vi "PathVelocityProfile.vi"(0 "Pose":dbl[](array[numeric]), 1 "time":dbl, 3 "intervalo":dbl=0.016, 5 "estimatives":T1, 9 "Path  Smooth":dbl[][](array[numeric]), 11 "V_max":dbl format="%#_13g", 13 "Accel":dbl=10.0, 14 "DesAccel":dbl=15.0) -> (4 "Time X":dbl[](array[numeric]), 6 "Velocities X":dbl[](array[numeric]), 8 "Time Y":dbl[](array[numeric]), 10 "Velocities Y":dbl[](array[numeric]))   [LabVIEW 2023]
uses:
  Controle/VelocityProfileState.ctl
  Controls/estimatives.ctl
  <vilib>/Analysis/_algsub.llb/Real Vector Norm.vi
  <vilib>/Analysis/coordinate.llb/Wrap Angle (scalar).vi
  <vilib>/Analysis/NI_AAL_Angle.lvlib
  <vilib>/Analysis/NI_AALPro.lvlib
panel:
  in  "est_vy":dbl
  in  "est_vx":dbl
  out "VelocityProfile Y":T2[](array[typedef])
  out "VelocityProfile X":T2[](array[typedef])
  out "Velocity Profile Y":cluster{dbl[], dbl[]}[](graph)
  out "Velocity Profile X":cluster{dbl[], dbl[]}[](graph)
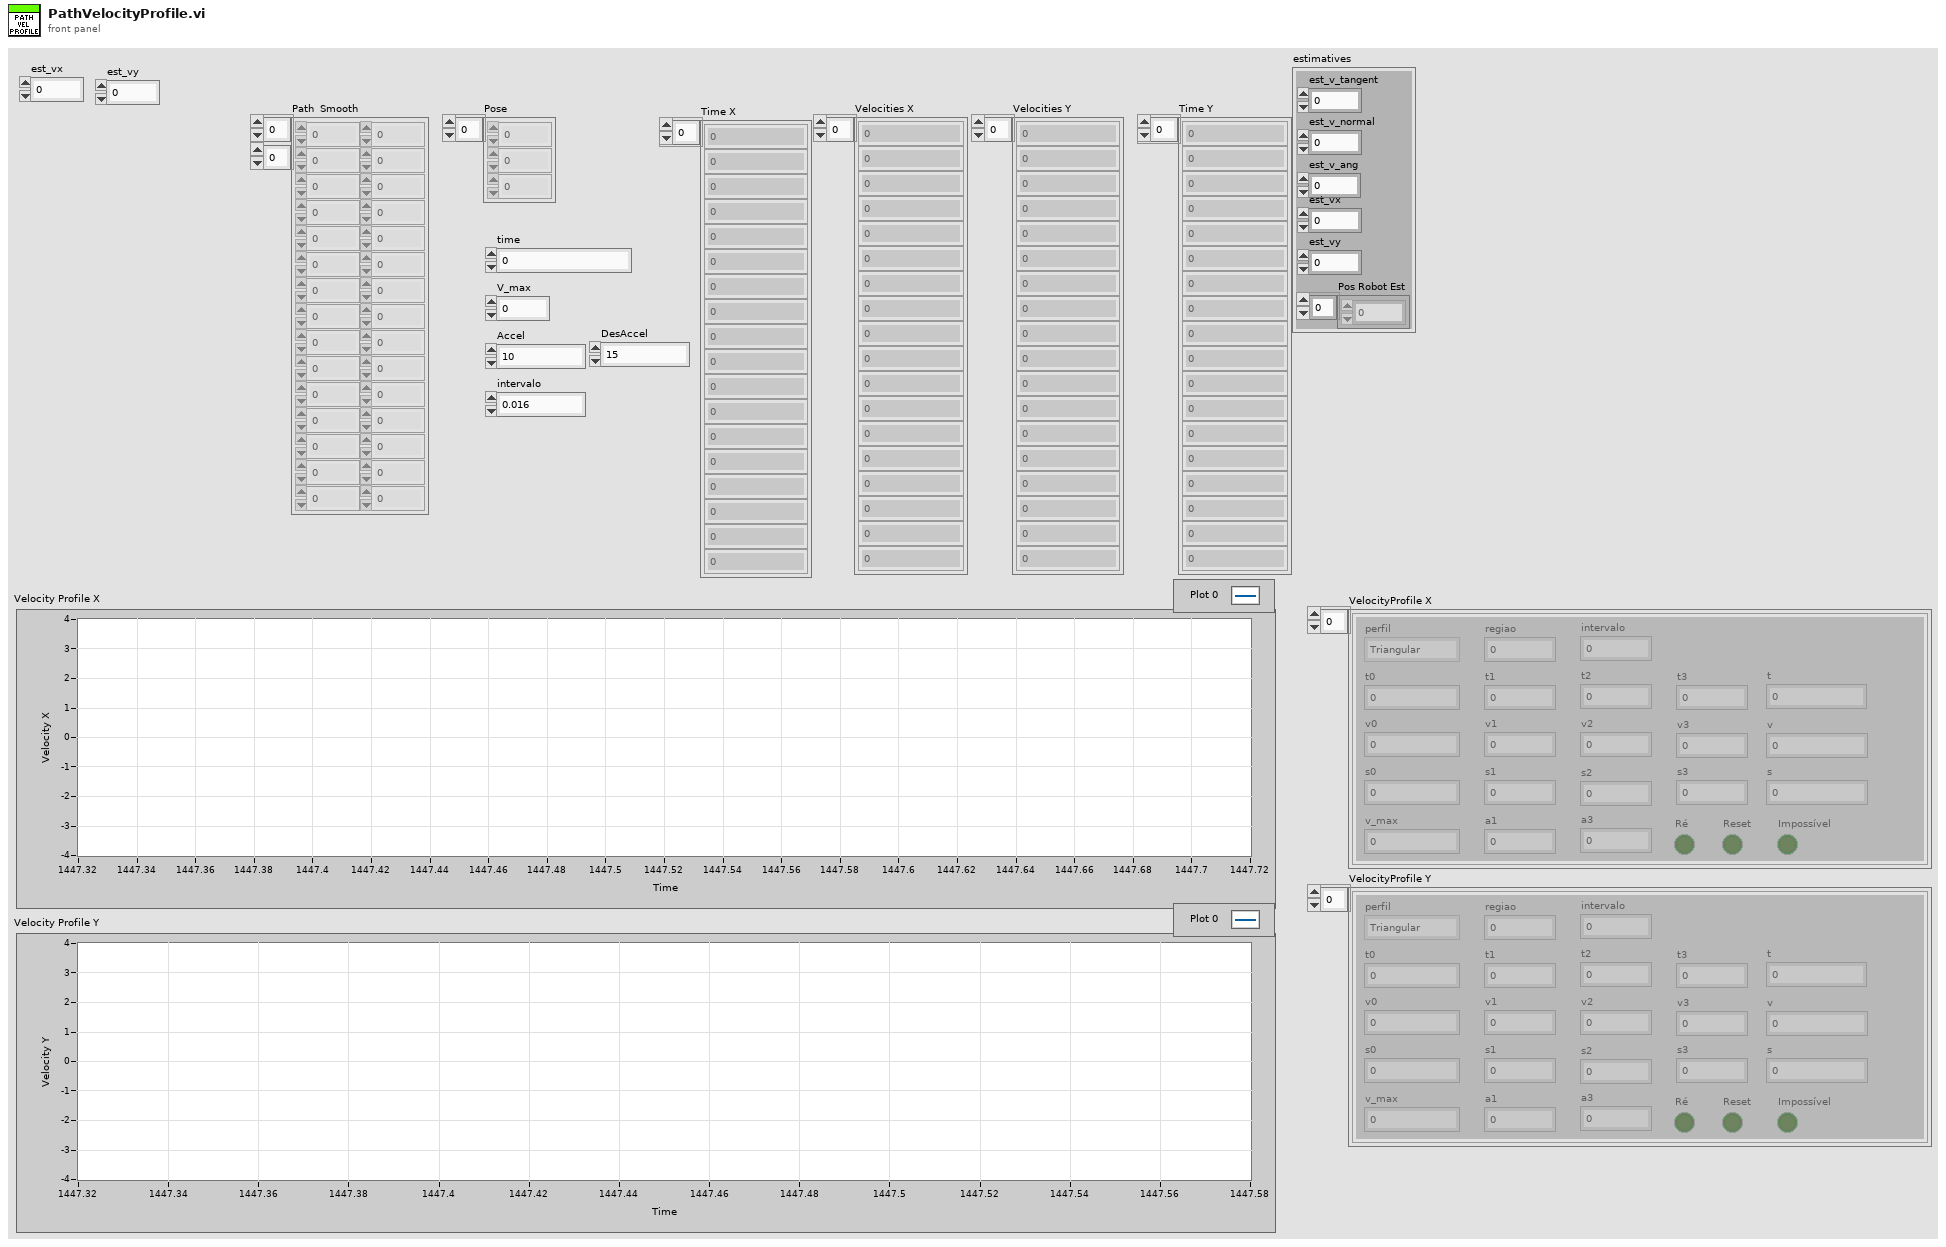
[diagram p1: front panel]
types:
  T1 = typedef "estimatives.ctl" = cluster{"est_v_tangent":dbl, "est_v_normal":dbl, "est_vx":dbl, "est_vy":dbl, "Pos Robot Est":dbl[], "est_v_ang":dbl}
  T2 = typedef "VelocityProfileState.ctl" = cluster{"t0":dbl, "t1":dbl, "t2":dbl, "t3":dbl, "v0":dbl, "v_max":dbl, "v3":dbl, "v2":dbl, "v1":dbl, "perfil":enum16{"Triangular", "Trapezoidal"}, "regiao":i32, "s0":dbl, "s1":dbl, "s2":dbl, "v":dbl, "t":dbl, "a1":dbl, "s3":dbl, "Reset":bool, "s":dbl, "a3":dbl, "Ré":bool, "Impossível":bool, "intervalo":dbl}
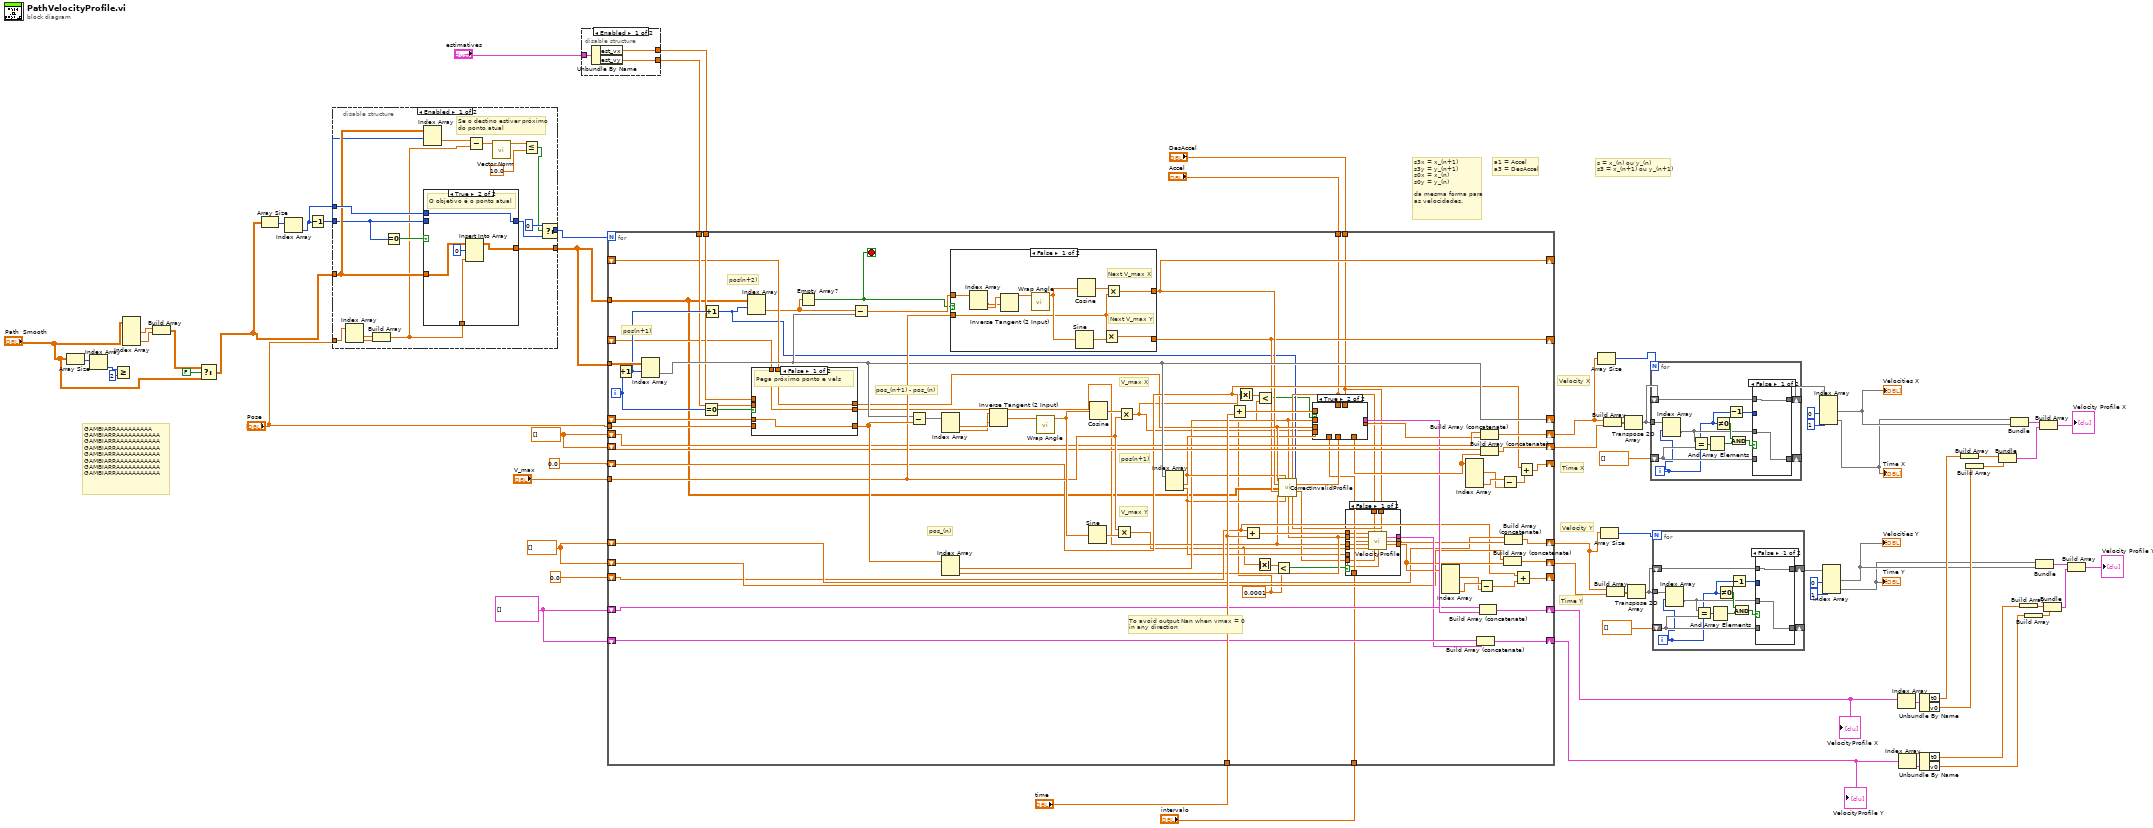
[diagram p0: block diagram]
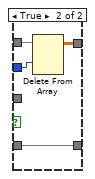
[diagram p4: hidden frame]
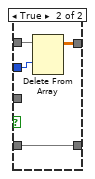
[diagram p5: hidden frame]
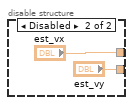
[diagram p6: hidden frame]
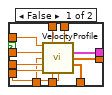
[diagram p7: hidden frame]
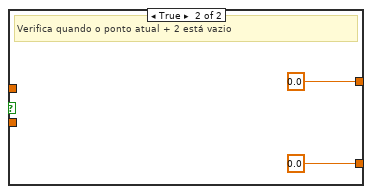
[diagram p9: hidden frame]
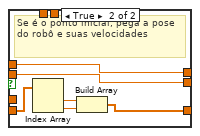
[diagram p10: hidden frame]
diagram:
  w57 = T2[] []
  w59 = dbl[] []
  w58 = dbl[] []
  # "GAMBIARRAAAAAAAAA \nGAMBIARRAAAAAAAAAAA\nGAMBIARRAAAAAAAAAAA\nGAMBIARRAAAAAAAAAAA\nGAMBIARRAAAAAAAAAAA\nGAMBIARRAAAAAAAAAAA\nGAMBIARRAAAAAAAAAAA\nGAMBIARRAAAAAAAAAAA"
  # "s = x_(n) ou y_(n)\ns3 = x_(n+1) ou y_(n+1)"
  # "a1 = Accel\na3 = DesAccel"
  # "s3x = x_(n+1)\ns3y = y_(n+1)\ns0x = x_(n)\ns0y = y_(n)\n\nda mesma forma para\nas velocidades."
  # "Time X"
  # "Time Y"
  # "Velocity Y"
  # "Velocity X"
  n1 = Array Size(array="Path  Smooth") -> (size(s)=w10:i32[])
  n2 = Index Array(array=w10) -> (element=w9:i32)  [unwired: 1 in]
  n3 = Greater Or Equal?(x=w9, y=2) -> ()  [unwired: 1 out]
  n4 = Index Array(array="Path  Smooth") -> (element #1=w6:dbl[], element #2=w5:dbl[])  [unwired: 4 in]
  n5 = Build Array(w6, w5) -> (w4:dbl[][])
  n6 = Select(t=w4, s=FALSE, f="Path  Smooth") -> (s? t:f=w3:dbl[][])
  n7 = Array Size(array=w3) -> (size(s)=w62:i32[])
  n8 = Index Array(array=w62) -> (element=w15:i32)  [unwired: 1 in]
  n9 = Decrement(x=w15) -> (x-1=w13:i32)
  n10 = disable-structure shown="Enabled" {
    disable-tunnel: [w85 w93] -> w12
    disable-tunnel: w15 -> [w83 _]
    disable-tunnel: "Pose" -> [w82 _]
    disable-tunnel: [w79 w94] -> w11
    disable-tunnel: w3 -> [w76 w93]
    disable-tunnel: w13 -> [w75 w94]
    frame Enabled {
      # "Se o destino estiver próximo\ndo ponto atual"
      n11 = Index Array(array=w82) -> (element #1=w81:dbl, element #2=w80:dbl)  [unwired: 2 in]
      n12 = Build Array(w81, w80) -> (w73:dbl[])
      n13 = Equal To 0?(x=w75) -> (x = 0?=w84:bool)
      n14 = Index Array(array=w76, index (row)=w75) -> (element=w74:dbl[])  [unwired: 1 in]
      n15 = case shown="True" w84 {
        tunnel: [w86 w88] -> w85
        tunnel: w76 -> [w86 w90]
        tunnel: [w87 w92] -> w78
        tunnel: w75 -> [w87 _]
        tunnel: w83 -> [_ w92]
        tunnel: w73 -> [_ w91]
        frame False {
          # "Passa o path para percorrer"
        }
        frame True {
          # "O objetivo é o ponto atual"
          n16 = Insert Into Array(array=w90, index (row)=0, new element=w91) -> (w88:dbl[][])  [unwired: 1 in]
        }
      }
      n17 = Subtract(x=w74, y=w73) -> (x-y=w72:dbl[])
      n18 = call-poly <vilib>:"Vector Norm.vi"("Input Vector"=w72) -> ("norm"=w71:dbl)  [unwired: 9 in, 1 out]
      n19 = Less Or Equal?(x=w71, y=10.0) -> (x <= y?=w69:bool)
      n20 = Select(t=0, s=w69, f=w78) -> (s? t:f=w79:i32)
    }
    frame Disabled {
    }
  }
  n21 = disable-structure shown="Enabled" {
    disable-tunnel: "estimatives" -> [w97 _]
    disable-tunnel: [w96 "est_vx"] -> w61
    disable-tunnel: [w95 "est_vy"] -> w60
    frame Enabled {
      n22 = Unbundle By Name(w97) -> ("est_vx"=w96:dbl, "est_vy"=w95:dbl)
    }
    frame Disabled {
    }
  }
  n23 = for {
    N: w11 -> [_]
    tunnel: w12 -> [w158]
    tunnel: "Pose" -> [w174]
    shift-right: [w159] -> _
    shift-left: _ -> [w173]
    tunnel: "V_max" -> [w163]
    tunnel: "Accel" -> [w113]
    tunnel: "DesAccel" -> [w112]
    tunnel: w12 -> [w109]
    shift-right: [w127] -> _
    shift-left: 0.0 ("t3") -> [w129]
    shift-right: [w125] -> _
    shift-left: 0.0 ("t3") -> [w124]
    tunnel: "time" -> [w161]
    shift-right: [w152] -> w36
    shift-left: w58 -> [w157]
    shift-right: [w155] -> w39
    shift-left: w58 -> [w156]
    shift-right: [w133] -> w18
    shift-left: w59 -> [w131]
    shift-right: [w132] -> w19
    shift-left: w59 -> [w130]
    tunnel: w61 -> [w149]
    tunnel: w60 -> [w148]
    shift-right: [w122] -> _
    shift-left: _ -> [w147]
    shift-right: [w116] -> _
    shift-left: _ -> [w146]
    shift-right: [w138] -> w55
    shift-left: w57 -> [w141]
    shift-right: [w137] -> w54
    shift-left: w57 -> [w140]
    tunnel: "intervalo" -> [w107]
    i -> [w110]
    stop <- w150 stop-if-true
    w101 = 0.0001 ("y")
    # "To avoid output Nan when vmax = 0\nin any direction"
    # "pos(n+2)"
    # "pos(n+1)"
    # "pos(n+1)"
    # "pos_(n)"
    # "pos_(n+1) - pos_(n)"
    # "V_max Y"
    # "V_max X"
    n24 = Increment(x=w110) -> (x+1=w154:i32)
    n25 = Index Array(array=w158, index (row)=w154) -> (element=w159:dbl[])  [unwired: 1 in]
    n26 = Equal To 0?(x=w110) -> (x = 0?=w175:bool)
    n27 = Increment(x=w154) -> (x+1=w108:i32)
    n28 = Index Array(array=w109, index (row)=w108) -> (element=w111:dbl[])  [unwired: 1 in]
    n29 = case shown="False" w175 {
      tunnel: w174 -> [_ w220]
      tunnel: [w214 w217] -> w165
      tunnel: w173 -> [w214 _]
      tunnel: w149 -> [_ w216]
      tunnel: w148 -> [_ w215]
      tunnel: [w212 w216] -> w123
      tunnel: [w213 w215] -> w118
      tunnel: w147 -> [w212 _]
      tunnel: w146 -> [w213 _]
      frame False {
        # "Pega próximo ponto e vels"
      }
      frame True {
        # "Se é o ponto inicial, pega a pose\ndo robô e suas velocidades"
        n30 = Index Array(array=w220) -> (element #1=w219:dbl, element #2=w218:dbl)  [unwired: 2 in]
        n31 = Build Array(w219, w218) -> (w217:dbl[])
      }
    }
    n32 = Empty Array?(array=w111) -> (empty?=w150:bool)
    n33 = Subtract(x=w111, y=w159) -> (x-y=w164:dbl[])
    n34 = Subtract(x=w159, y=w165) -> (x-y=w171:dbl[])
    n35 = Index Array(array=w171) -> (element #1=w172:dbl, element #2=w170:dbl)  [unwired: 2 in]
    n36 = Index Array(array=w165) -> (element #1=w120:dbl, element #2=w119:dbl)  [unwired: 2 in]
    n37 = case shown="False" w150 {
      tunnel: w164 -> [w204 _]
      tunnel: w163 -> [w202 _]
      tunnel: [w201 0.0] -> w122
      tunnel: [w200 0.0] -> w116
      frame False {
        # "Next V_max Y"
        # "Next V_max X"
        n38 = Index Array(array=w204) -> (element #1=w203:dbl, element #2=w205:dbl)  [unwired: 2 in]
        n39 = Inverse Tangent (2 Input)(1:w203, 2:w205) -> (0:w206:dbl)
        n40 = call-poly <vilib>:"Wrap Angle.vi"("angle in"=w206) -> ("angle out"=w207:dbl)  [unwired: 9 in, 1 out]
        n41 = Sine(x=w207) -> (sin(x)=w209:dbl)
        n42 = Cosine(x=w207) -> (cos(x)=w208:dbl)
        n43 = Multiply(x=w202, y=w209) -> (x*y=w200:dbl)
        n44 = Multiply(x=w208, y=w202) -> (x*y=w201:dbl)
      }
      frame True {
        # "Verifica quando o ponto atual + 2 está vazio"
      }
    }
    n45 = Inverse Tangent (2 Input)(1:w172, 2:w170) -> (0:w169:dbl)
    n46 = call-poly <vilib>:"Wrap Angle.vi"("angle in"=w169) -> ("angle out"=w168:dbl)  [unwired: 9 in, 1 out]
    n47 = Sine(x=w168) -> (sin(x)=w166:dbl)
    n48 = Cosine(x=w168) -> (cos(x)=w167:dbl)
    n49 = Multiply(x=w163, y=w166) -> (x*y=w106:dbl)
    n50 = Multiply(x=w167, y=w163) -> (x*y=w102:dbl)
    n51 = Index Array(array=w159) -> (element #1=w121:dbl, element #2=w117:dbl)  [unwired: 2 in]
    n52 = Add(x=w129, y=w161) -> (x+y=w162:dbl)
    n53 = Absolute Value(x=w102) -> (abs(x)=w103:dbl)
    n54 = Add(x=w124, y=w161) -> (x+y=w160:dbl)
    n55 = Absolute Value(x=w106) -> (abs(x)=w105:dbl)
    n56 = Less?(x=w103, y=w101) -> (x < y?=w100:bool)
    n57 = Less?(x=w105, y=w101) -> (x < y?=w104:bool)
    n58 = call "CorrectInvalidProfile.vi"("v0x"=w123, "s3x"=w121, "s0x"=w120, "a1"=w113, "index"=w108, "v3x"=w122, "Path  Smooth"=w109, "v3y"=w116, "v0y"=w118, "s3y"=w117, "s0y"=w119, "a3"=w112) -> ("New v3x"=w114:dbl, "New v3y"=w115:dbl)  [unwired: 2 in]
    n59 = case shown="True" w100 {
      tunnel: w102 -> [w187 _]
      tunnel: w162 -> [w186 _]
      tunnel: [w185 _] -> w153
      tunnel: [w184 _] -> w151
      tunnel: [w183 _] -> w142
      tunnel: w123 -> [w182 _]
      tunnel: w121 -> [w181 _]
      tunnel: w120 -> [w180 _]
      tunnel: w114 -> [w179 _]
      tunnel: w113 -> [w178 _]
      tunnel: w112 -> [w177 _]
      tunnel: w107 -> [w176 _]
      frame False {
        n60 = call "VelocityProfile.vi"("t"=w186, "a1"=w178, "a3"=w177, "s"=w180, "intervalo"=w176, "v_est"=w182, "v_max"=w187, "v3"=w179, "s3"=w181) -> ("VelocityProfileState Out"=w183:T2, "Velocities"=w185:dbl[], "Time"=w184:dbl[])  [unwired: 3 in, 1 out]
      }
      frame True {
      }
    }
    n61 = case shown="False" w104 {
      tunnel: w106 -> [w199 _]
      tunnel: w160 -> [w198 _]
      tunnel: [w197 _] -> w139
      tunnel: [w196 _] -> w136
      tunnel: [w195 _] -> w134
      tunnel: w119 -> [w194 _]
      tunnel: w118 -> [w193 _]
      tunnel: w117 -> [w192 _]
      tunnel: w115 -> [w191 _]
      tunnel: w113 -> [w190 _]
      tunnel: w112 -> [w189 _]
      tunnel: w107 -> [w188 _]
      frame False {
        n62 = call "VelocityProfile.vi"("t"=w198, "a1"=w190, "a3"=w189, "s"=w194, "intervalo"=w188, "v_est"=w193, "v_max"=w199, "v3"=w191, "s3"=w192) -> ("VelocityProfileState Out"=w197:T2, "Velocities"=w196:dbl[], "Time"=w195:dbl[])  [unwired: 3 in, 1 out]
      }
      frame True {
      }
    }
    n63 = Index Array(array=w134) -> (element #1=w144:dbl, element #4=w145:dbl)  [unwired: 4 in, 2 out]
    n64 = Index Array(array=w151) -> (element #1=w135:dbl, element #4=w143:dbl)  [unwired: 4 in, 2 out]
    n65 = Build Array (concatenate)(w140, w139) -> (w137:T2[])
    n66 = Subtract(x=w145, y=w144) -> (x-y=w126:dbl)
    n67 = Build Array (concatenate)(w141, w142) -> (w138:T2[])
    n68 = Build Array (concatenate)(w157, w153) -> (w152:dbl[])
    n69 = Build Array (concatenate)(w156, w151) -> (w155:dbl[])
    n70 = Subtract(x=w143, y=w135) -> (x-y=w128:dbl)
    n71 = Build Array (concatenate)(w130, w134) -> (w132:dbl[])
    n72 = Build Array (concatenate)(w131, w136) -> (w133:dbl[])
    n73 = Add(x=w124, y=w126) -> (x+y=w125:dbl)
    n74 = Add(x=w129, y=w128) -> (x+y=w127:dbl)
  }
  "VelocityProfile X" <- w55
  "VelocityProfile Y" <- w54
  n75 = Array Size(array=w36) -> (size(s)=w33:i32)
  n76 = Array Size(array=w18) -> (size(s)=w22:i32)
  n77 = Build Array(w36, w39) -> (w32:dbl[][])
  n78 = Build Array(w18, w19) -> (w23:dbl[][])
  n79 = Transpose 2D Array(2D array=w32) -> (transposed array=w31:dbl[][])
  n80 = Transpose 2D Array(2D array=w23) -> (transposed array=w24:dbl[][])
  n81 = for {
    N: w33 -> [_]
    tunnel: w31 -> [w224]
    shift-right: [w232] -> _
    shift-left: dbl[] [] -> [w231]
    shift-right: [w225] -> w34
    shift-left: w31 -> [w226]
    i -> [w221]
    n82 = Index Array(array=w224, index (row)=w221) -> (element=w223:dbl[])  [unwired: 1 in]
    n83 = Equal?(x=w223, y=w231) -> (x = y?=w230:bool[])
    n84 = And Array Elements(Boolean array=w230) -> (logical AND=w229:bool)
    n85 = Not Equal To 0?(x=w221) -> (x != 0?=w228:bool)
    n86 = Decrement(x=w221) -> (x-1=w222:i32)
    n87 = And(x=w228, y=w229) -> (x .and. y?=w227:bool)
    n88 = case shown="False" w227 {
      tunnel: w223 -> [w234 _]
      tunnel: [w234 w238] -> w232
      tunnel: w231 -> [_ w238]
      tunnel: w226 -> [w233 w237]
      tunnel: [w233 w236] -> w225
      tunnel: w222 -> [_ w235]
      frame False {
      }
      frame True {
        n89 = Delete From Array(array=w237, index (row)=w235) -> (array with subset deleted=w236:dbl[][])  [unwired: 2 in, 1 out]
      }
    }
  }
  n90 = for {
    N: w22 -> [_]
    tunnel: w24 -> [w242]
    shift-right: [w250] -> _
    shift-left: dbl[] [] -> [w249]
    shift-right: [w243] -> w21
    shift-left: w24 -> [w244]
    i -> [w239]
    n91 = Index Array(array=w242, index (row)=w239) -> (element=w241:dbl[])  [unwired: 1 in]
    n92 = Equal?(x=w241, y=w249) -> (x = y?=w248:bool[])
    n93 = And Array Elements(Boolean array=w248) -> (logical AND=w247:bool)
    n94 = Not Equal To 0?(x=w239) -> (x != 0?=w246:bool)
    n95 = Decrement(x=w239) -> (x-1=w240:i32)
    n96 = And(x=w246, y=w247) -> (x .and. y?=w245:bool)
    n97 = case shown="False" w245 {
      tunnel: w241 -> [w252 _]
      tunnel: [w252 w256] -> w250
      tunnel: w249 -> [_ w256]
      tunnel: w244 -> [w251 w255]
      tunnel: [w251 w254] -> w243
      tunnel: w240 -> [_ w253]
      frame False {
      }
      frame True {
        n98 = Delete From Array(array=w255, index (row)=w253) -> (array with subset deleted=w254:dbl[][])  [unwired: 2 in, 1 out]
      }
    }
  }
  n99 = Index Array(array=w34, index (col) #1=0 ("disabled index (col)"), index (col) #2=1 ("index (col)")) -> (element #1=w38:dbl[], element #2=w37:dbl[])  [unwired: 2 in]
  "Velocities X" <- w38
  "Time X" <- w37
  n100 = Index Array(array=w21, index (col) #1=0 ("disabled index (col)"), index (col) #2=1 ("index (col)")) -> (element #1=w17:dbl[], element #2=w16:dbl[])  [unwired: 2 in]
  "Velocities Y" <- w17
  "Time Y" <- w16
  n101 = Index Array(array=w55) -> (element=w53:T2)  [unwired: 1 in]
  n102 = Index Array(array=w54) -> (element=w52:T2)  [unwired: 1 in]
  n103 = Unbundle By Name(w53) -> ("t0"=w45:dbl, "v0"=w44:dbl)
  n104 = Unbundle By Name(w52) -> ("t0"=w41:dbl, "v0"=w40:dbl)
  n105 = Build Array(w45) -> (w46:dbl[])
  n106 = Build Array(w44) -> (w47:dbl[])
  n107 = Bundle(w46, w47) -> (w27:cluster{dbl[], dbl[]})  [unwired: 1 in]
  n108 = Bundle(w37, w38) -> (w51:cluster{dbl[], dbl[]})  [unwired: 1 in]
  n109 = Build Array(w41) -> (w42:dbl[])
  n110 = Build Array(w40) -> (w43:dbl[])
  n111 = Bundle(w16, w17) -> (w49:cluster{dbl[], dbl[]})  [unwired: 1 in]
  n112 = Build Array(w51, w27) -> (→"Velocity Profile X":cluster{dbl[], dbl[]}[])
  n113 = Bundle(w42, w43) -> (w28:cluster{dbl[], dbl[]})  [unwired: 1 in]
  n114 = Build Array(w49, w28) -> (→"Velocity Profile Y":cluster{dbl[], dbl[]}[])
